vi "parse load from string.vi"(8 "error in":errorcluster, 11 "message data":string) -> (0 "error out":errorcluster, 2 "target index":i32, 3 "system data":string)   [LabVIEW 2013, in "module execution process.lvlib"]
uses:
  module execution process.lvlib
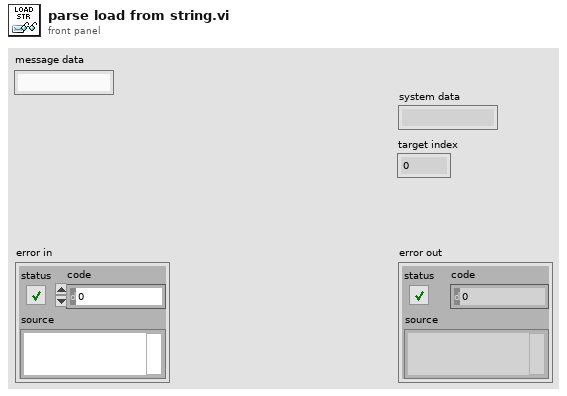
[diagram p1: front panel]
types:
  T1 = cluster{"system data":string, "target index":i32}
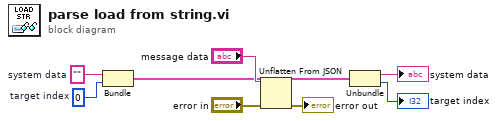
[diagram p0: block diagram]
diagram:
  w2 = 0  # target index
  w6 = ""  # system data
  n1 = Bundle("system data"=w6, "target index"=w2) -> (w5:T1)  [unwired: 1 in]
  n2 = Unflatten From JSON(JSON string="message data", type and defaults=w5, error in (no error)="error in") -> (value=w4:T1, error out=→"error out":errorcluster)  [unwired: 4 in]
  n3 = Unbundle(w4) -> ("system data"=→"system data":string, "target index"=→"target index":i32)
